vi "sub vi - Manual Phase Sweep.vi"(0 "Axis":u16(ring)=2 items=["X", "Y", "Z"], 1 "filename":string, 2 "# of Cycles":dbl=1.0 min=1.0 max=100.0 step=1.0, 5 "Desired Frequency":dbl=0.5 format="%.2f", 7 "Rate (Hz)":dbl=2500.0 format="%0.2f", 9 "Start":dbl, 11 "Low":dbl, 12 "High":dbl, 13 "Save Data":bool) -> (4 "# of Samples":dbl, 6 "Displacement vs Position":cluster{dbl[], dbl[]}[](graph), 8 "Waveform Graph":waveform(dbl)[](graph), 10 "correctV":dbl[](array[numeric]), 15 "Displacement vs Position 2":cluster{dbl[], dbl[]}[](graph))   [LabVIEW 2010]
uses:
  <vilib>/DAQmx/write.llb/DAQmx Write (Analog Wfm 1Chan NSamp).vi
  <vilib>/DAQmx/read.llb/DAQmx Read (Analog 1D Wfm NChan NSamp).vi
  <vilib>/DAQmx/create/channels.llb/DAQmx Create Channel (AI-Voltage-Basic).vi
  <vilib>/DAQmx/configure/timing.llb/DAQmx Timing (Sample Clock).vi
  <vilib>/DAQmx/create/channels.llb/DAQmx Create Channel (AO-Voltage-Basic).vi
  <vilib>/DAQmx/configure/timing.llb/DAQmx Timing (Use Waveform).vi
  <vilib>/daqmx/miscellaneous.llb/DAQmx Fill In Error Info.vi
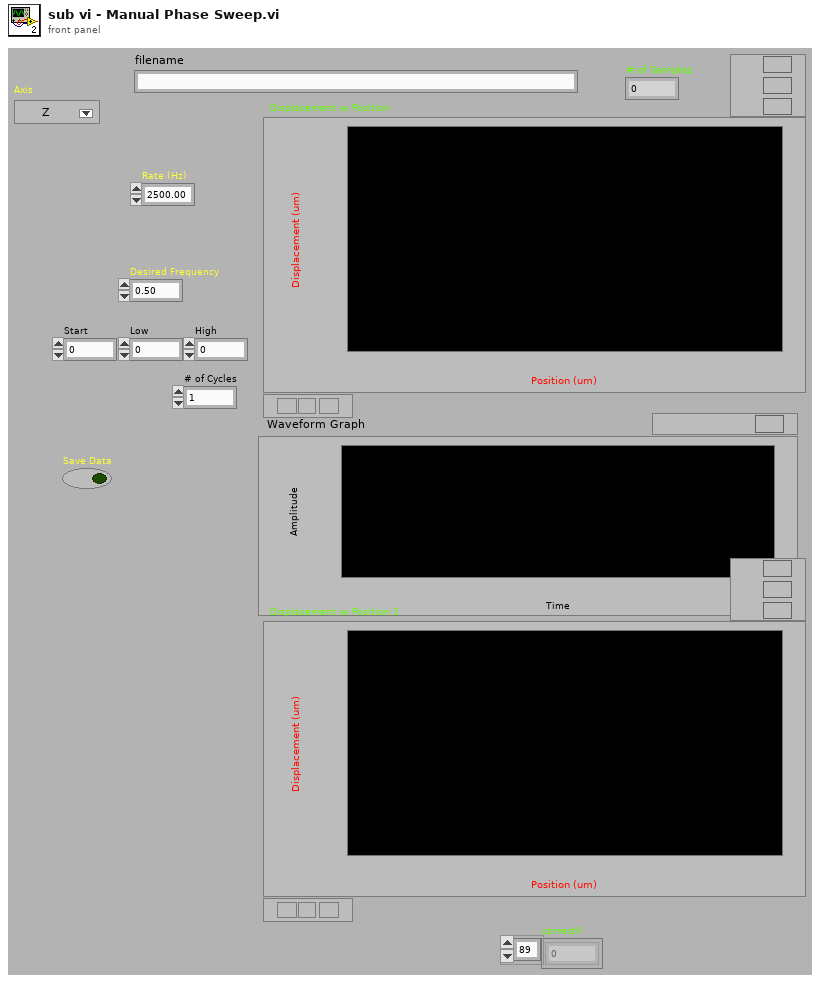
[diagram p1: front panel]
types:
  T1 = cluster{"Waveform":waveform(dbl), "Waveform":waveform(dbl)}
  T2 = cluster{"Waveform":waveform(dbl), "Waveform":waveform(dbl)}[]
  T3 = cluster{waveform(dbl), "Waveform":waveform(dbl)}[]
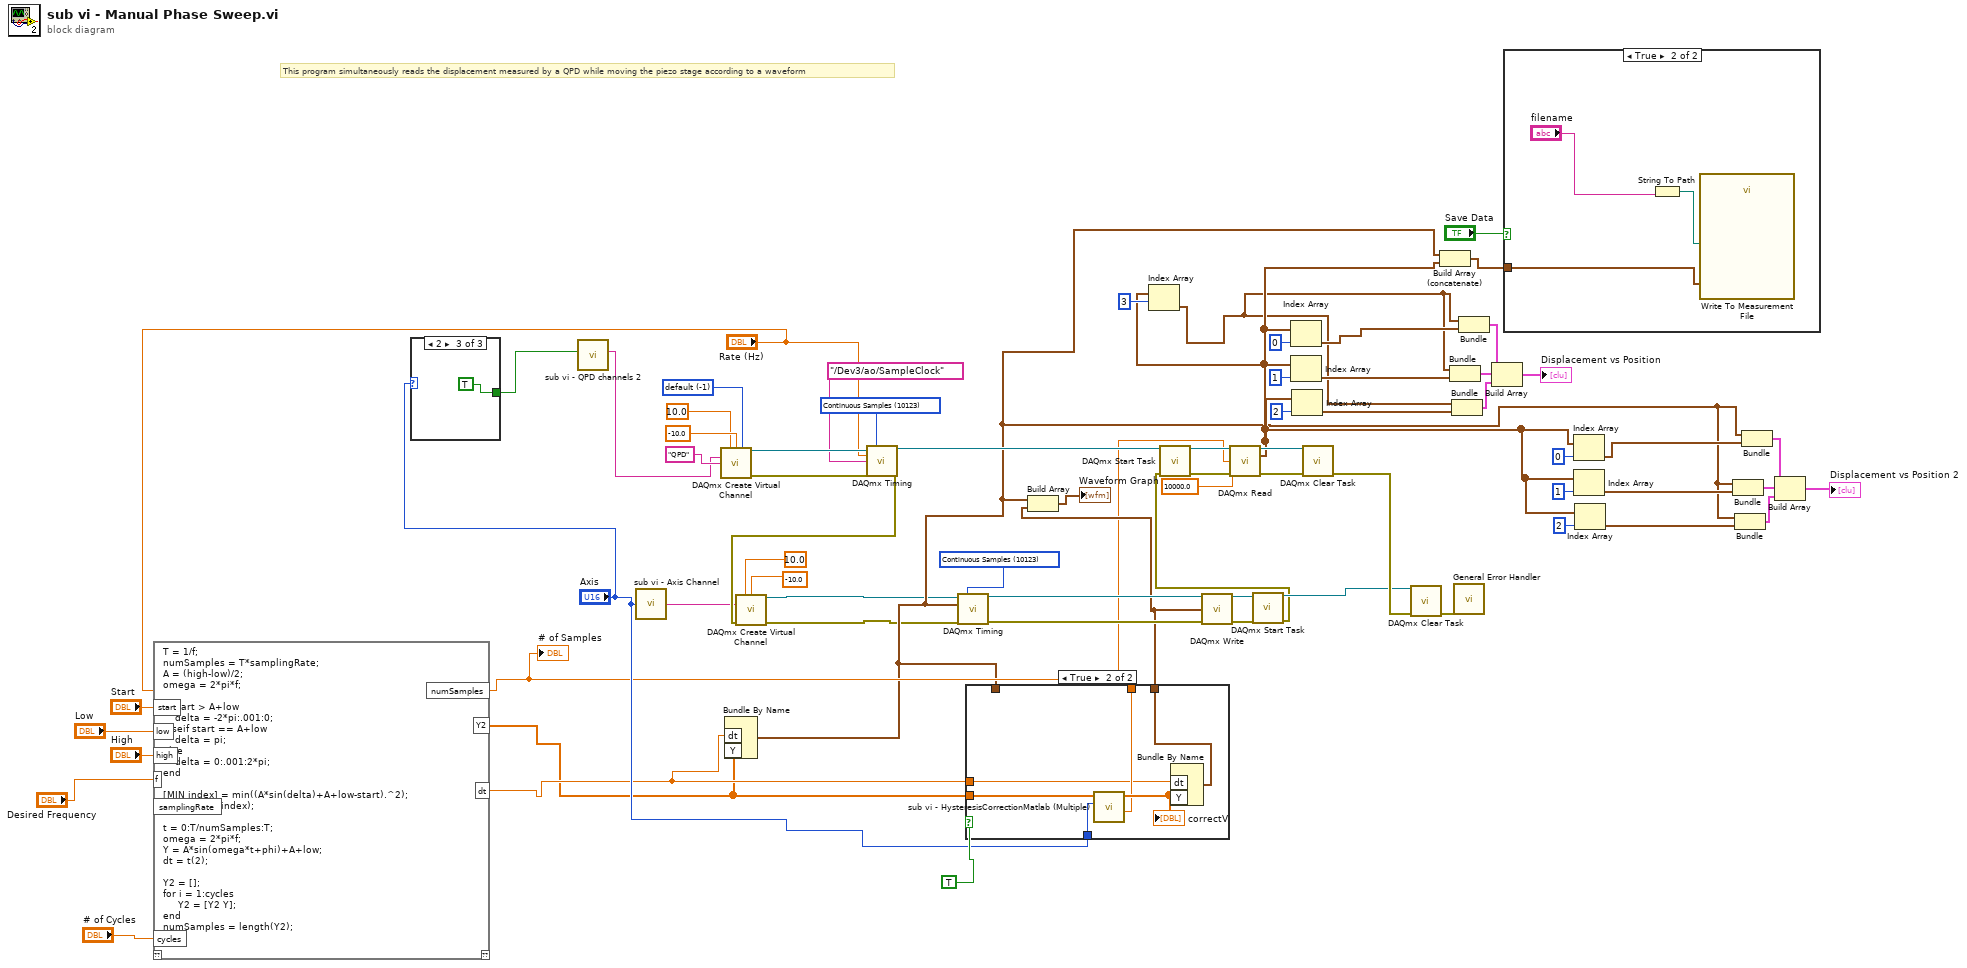
[diagram p0: block diagram]
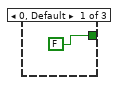
[diagram p2: hidden frame]
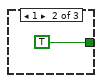
[diagram p3: hidden frame]
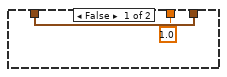
[diagram p5: hidden frame]
diagram:
  w55 = -1 items=["default"=-1, "RSE"=10083, "NRSE"=10078, "Differential"=10106, "Pseudodifferential"=12529] ("input terminal configuration")
  w60 = 10123 items=["Finite Samples"=10178, "Continuous Samples"=10123, "Hardware Timed Single Point"=12522] ("sample mode")
  w67 = 10123 items=["Finite Samples"=10178, "Continuous Samples"=10123, "Hardware Timed Single Point"=12522] ("sample mode")
  # "This program simultaneously reads the displacement measured by a QPD while moving the piezo stage according to a waveform"
  n1 = script code="T = 1/f;\nnumSamples = T*samplingRate;\nA = (high-low)/2;\nomega = 2*pi*f;\n\nif start > A+low\n    delta = -2*pi:.001:0;\nelseif start == A+low\n    delta = pi;\nelse\n    delta = 0:.001:2*pi;\nend\n\n[MIN index] = min((A*sin(delta)+A+low-start).^2);\nphi = delta(index);\n\nt = 0:T/numSamples:T;\nomega = 2*pi*f;\nY = A*sin(omega*t+phi)+A+low;\ndt = t(2);\n\nY2 = [];\nfor i = 1:cycles\n     Y2 = [Y2 Y];\nend\nnumSamples = length(Y2);"("start"="Start", "low"="Low", "high"="High", "f"="Desired Frequency", "samplingRate"="Rate (Hz)", "cycles"="# of Cycles") -> ("Y2"=w6:dbl[], "dt"=w7:dbl, "numSamples"=w9:dbl)  [unwired: 1 in, 1 out]
  "# of Samples" <- w9
  n2 = case shown="2" "Axis" {
    tunnel: [FALSE ("Include Position?") TRUE ("Include Position?") TRUE ("Include Position?")] -> w16
    frame 0, Default {
    }
    frame 1 {
    }
    frame 2 {
    }
  }
  n3 = call "sub vi - QPD channels 2.vi"("Include Position?"=w16) -> ("QPD Channels"=w35:tag)  [unwired: 9 out]
  n4 = call "sub vi - Axis Channel.vi"("Axis"="Axis") -> ("physical channels"=w54:tag)
  n5 = call-poly <vilib>:"DAQmx Create Virtual Channel.vi"("maximum value"=10.0, "minimum value"=-10.0, "input terminal configuration"=w55, "physical channels"=w35, "name to assign"="QPD") -> ("task out"=w70:refnum<k21>, "error out"=w69:errorcluster)  [unwired: 4 in, 5 out]
  n6 = Bundle By Name("dt"=w7, "Y"=w6) -> (w5:waveform(dbl))  [unwired: 1 out]
  n7 = call-poly <vilib>:"DAQmx Timing.vi"("task/channels in"=w70, "sample mode"=w67, "rate"="Rate (Hz)", "source"=tag "/Dev3/ao/SampleClock", "error in"=w69) -> ("task out"=w66:refnum<k21>, "error out"=w64:errorcluster)  [unwired: 2 in, 7 out]
  n8 = call-poly <vilib>:"DAQmx Create Virtual Channel.vi"("maximum value"=10.0, "minimum value"=-10.0, "physical channels"=w54, "error in"=w64) -> ("task out"=w4:refnum<k21>, "error out"=w3:errorcluster)  [unwired: 5 in, 5 out]
  n9 = call-poly <vilib>:"DAQmx Timing.vi"("task/channels in"=w4, "sample mode"=w60, "waveform"=w5, "error in"=w3) -> ("task out"=w61:refnum<k21>, "error out"=w62:errorcluster)  [unwired: 1 in, 9 out]
  n10 = case shown="True" TRUE {
    tunnel: w5 -> [w75 _]
    tunnel: [w75 w81] -> w30
    tunnel: "Axis" -> [_ w80]
    tunnel: [1.0 ("Strain2um") w78] -> _
    tunnel: w6 -> [_ w77]
    tunnel: w7 -> [_ w76]
    frame False {
    }
    frame True {
      n11 = call "sub vi - HysteresisCorrectionMatlab (Multiple).vi"("Axis"=w80, "desired positions"=w77) -> ("Strain2um"=w78:dbl, "correctV"=w79:dbl[])  [unwired: 2 in, 6 out]
      "correctV" <- w79
      n12 = Bundle By Name("dt"=w76, "Y"=w79) -> (w81:waveform(dbl))  [unwired: 1 out]
    }
  }
  n13 = Build Array(w5, w30) -> (→"Waveform Graph":waveform(dbl)[])
  n14 = call-poly <vilib>:"DAQmx Write.vi"("task/channels in"=w61, "data"=w30, "error in"=w62) -> ("task out"=w37:refnum<k21>, "error out"=w36:errorcluster)  [unwired: 1 in, 10 out]
  n15 = call <vilib>:"DAQmx Start Task.vi"("task/channels in"=w37, "error in"=w36) -> ("task out"=w52:refnum<k21>, "error out"=w40:errorcluster)  [unwired: 12 out]
  n16 = call <vilib>:"DAQmx Start Task.vi"("task/channels in"=w66, "error in"=w40) -> ("task out"=w39:refnum<k21>, "error out"=w38:errorcluster)  [unwired: 12 out]
  n17 = call-poly <vilib>:"DAQmx Read.vi"("task/channels in"=w39, "number of samples per channel"=w9, "timeout"=10000.0, "error in"=w38) -> ("task out"=w42:refnum<k21>, "data"=w20:waveform(dbl)[], "error out"=w41:errorcluster)  [unwired: 9 out]
  n18 = Index Array(array=w20, index=3) -> (element=w14:waveform(dbl))
  n19 = Index Array(array=w20, index=0) -> (element=w34:waveform(dbl))
  n20 = Index Array(array=w20, index=1) -> (element=w45:waveform(dbl))
  n21 = Index Array(array=w20, index=2) -> (element=w44:waveform(dbl))
  n22 = call <vilib>:"DAQmx Clear Task.vi"("task in"=w42, "error in"=w41) -> ("error out"=w53:errorcluster)  [unwired: 13 out]
  n23 = call <vilib>:"DAQmx Clear Task.vi"("task in"=w52, "error in"=w53) -> ("error out"=w63:errorcluster)  [unwired: 13 out]
  n24 = Build Array (concatenate)(w5, w20) -> (w32:waveform(dbl)[])
  n25 = Bundle("Waveform"=w14, "Waveform"=w45) -> (w46:T1)  [unwired: 1 out]
  n26 = Bundle("Waveform"=w14, "Waveform"=w44) -> (w47:T1)  [unwired: 1 out]
  n27 = call <vilib>:"General Error Handler.vi"("error in (no error)"=w63) -> ()  [unwired: 2 in, 13 out]
  n28 = Bundle("Waveform"=w14, "Waveform"=w34) -> (w48:T1)  [unwired: 1 out]
  n29 = Build Array(w48, w46, w47) -> (→"Displacement vs Position":T2)
  n30 = case shown="True" "Save Data" {
    tunnel: w32 -> [_ w83]
    frame False {
    }
    frame True {
      n31 = String To Path(string="filename") -> (path=w84:path)
      n32 = call "Write To Measurement File"("Signals"=w83, "Filename"=w84) -> ()  [unwired: 15 in, 3 out]
    }
  }
  n33 = Index Array(array=w20, index=0) -> (element=w19:waveform(dbl))
  n34 = Index Array(array=w20, index=1) -> (element=w22:waveform(dbl))
  n35 = Index Array(array=w20, index=2) -> (element=w21:waveform(dbl))
  n36 = Bundle(w5, "Waveform"=w22) -> (w23:cluster{waveform(dbl), "Waveform":waveform(dbl)})  [unwired: 1 out]
  n37 = Bundle(w5, "Waveform"=w21) -> (w24:cluster{waveform(dbl), "Waveform":waveform(dbl)})  [unwired: 1 out]
  n38 = Bundle(w5, "Waveform"=w19) -> (w25:cluster{waveform(dbl), "Waveform":waveform(dbl)})  [unwired: 1 out]
  n39 = Build Array(w25, w23, w24) -> (→"Displacement vs Position 2":T3)
